vi "asset.get_from_datasouce.path.vi"(8 "error in":errorcluster, 10 "datasource rid":string) -> (0 "error out":errorcluster, 3 "path":string)   [LabVIEW 2020, in "Nominal Client.lvclass"]
uses:
  Nominal Client.lvclass
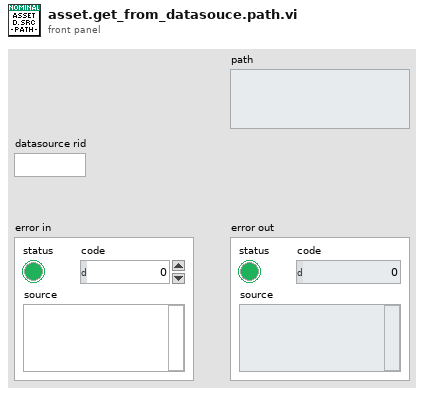
[diagram p1: front panel]
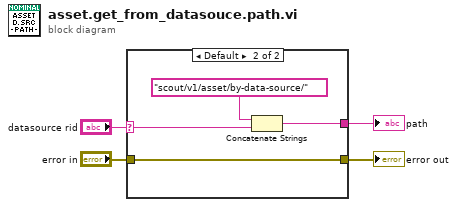
[diagram p0: block diagram]
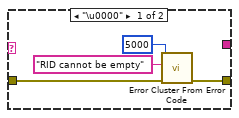
[diagram p2: hidden frame]
diagram:
  n1 = case shown="Default" "datasource rid" {
    selector: "datasource rid" -> [_ w11]
    tunnel: [_ w10] -> w3
    tunnel: "error in" -> [w5 w9]
    tunnel: [w6 w9] -> w1
    frame "\u0000" {
      n2 = call <vilib>:"Error Cluster From Error Code.vi"("error in (no error)"=w5, "error message (\"\")"="RID cannot be empty" ("error message (\"\")"), "error code (0)"=5000) -> ("error out"=w6:errorcluster)  [unwired: 6 in]
    }
    frame Default {
      n3 = Concatenate Strings("scout/v1/asset/by-data-source/" ("Path"), w11) -> (w10:string)
    }
  }
  "path" <- w3
  "error out" <- w1
